vi "write outputs.vi"(10 "model outputs":T2, 11 "outputs":T1[](array[typedef]) format="%.0x") -> (0 "code":i32)   [LabVIEW 2015, in "Scriptable Model Interface Engine.lvlib"]
uses:
  Scriptable Model Interface Engine.lvlib
  Shared/model outputs.ctl
  <vilib>/NI Veristand/Custom Device API/Data Reference.ctl
  <vilib>/NI Veristand/Custom Device API/Global Data Refs.vi
  <vilib>/NI Veristand/Custom Device API/Custom Device API.lvlib
  Shared/Scriptable Model Interface Shared.lvlib
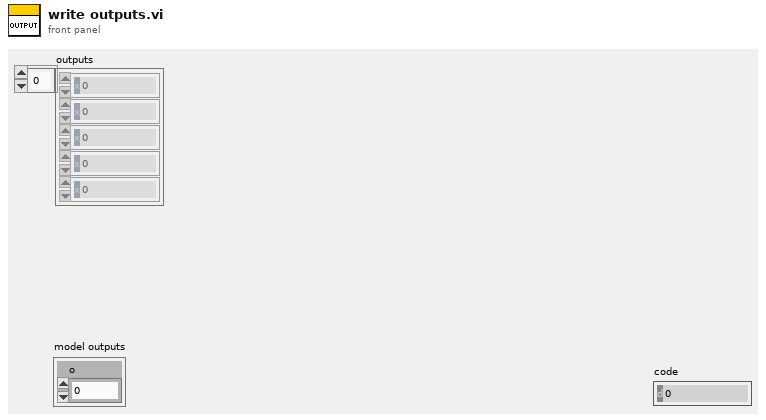
[diagram p1: front panel]
types:
  T1 = typedef "Custom Device API.lvlib/Data Reference.ctl" = i32
  T2 = typedef "Scriptable Model Interface Shared.lvlib/model outputs.ctl" = cluster{"o":dbl}
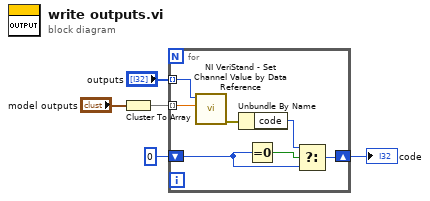
[diagram p0: block diagram]
diagram:
  n1 = Cluster To Array(cluster="model outputs") -> (array=w3:dbl[])
  n2 = for {
    tunnel: "outputs" -> [w12] mode=indexing
    tunnel: w3 -> [w11] mode=indexing
    shift-right: [w7] -> w2
    shift-left: 0 ("code") -> [w6]
    n3 = call <vilib>:"NI VeriStand - Set Channel Value by Data Reference.vi"("Value"=w11, "Data Reference in"=w12) -> ("error out"=w10:errorcluster)  [unwired: 9 in]
    n4 = Unbundle By Name(w10) -> ("code"=w8:i32)
    n5 = Equal To 0?(x=w6) -> (x = 0?=w9:bool)
    n6 = Select(t=w8, s=w9, f=w6) -> (s? t:f=w7:i32)
  }
  "code" <- w2
